vi "ParseArgumentsCore.vi"(8 "error in (no error)":errorcluster, 10 "Inputs":string[](array[string]), 11 "RunVIAnalyzer in":refnum<class "RunVIAnalyzer.lvclass">) -> (0 "error out":errorcluster, 3 "RunVIAnalyzer out":refnum<class "RunVIAnalyzer.lvclass">)   [LabVIEW 2018, in "RunVIAnalyzer.lvclass"]
uses:
  RunVIAnalyzer.lvclass
  RunVIAnalyzer.lvclass/RunVIAnalyzer.ctl
  Utilities/OperationErrorType.ctl
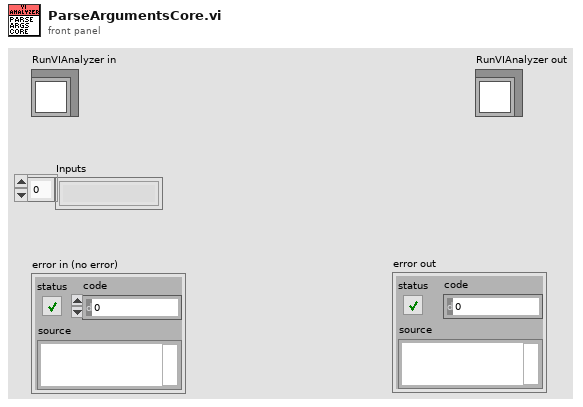
[diagram p1: front panel]
types:
  T1 = typedef "OperationErrorType.ctl" = enum16{"RequiredArgumentMissing", "UnknownArguments", "LoggerSetMultipleTimes", "OperationBrokenError"}
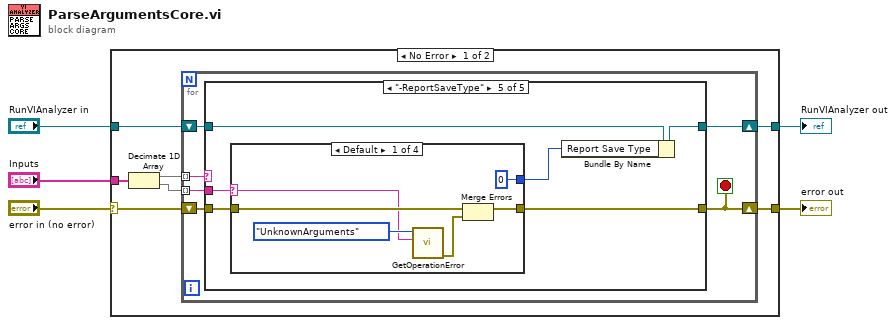
[diagram p0: block diagram]
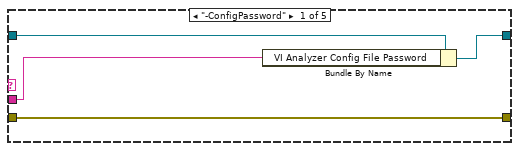
[diagram p2: hidden frame]
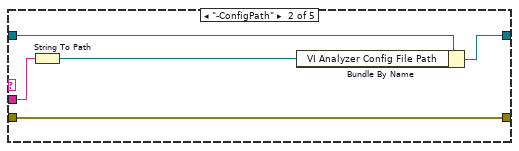
[diagram p3: hidden frame]
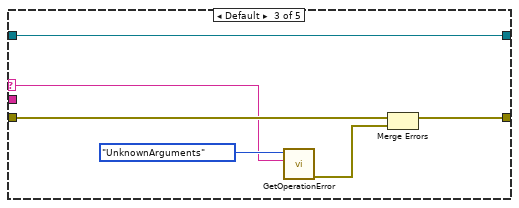
[diagram p4: hidden frame]
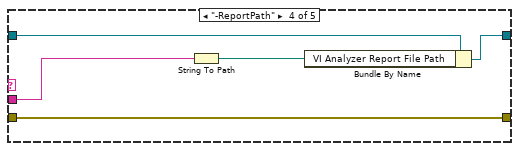
[diagram p5: hidden frame]
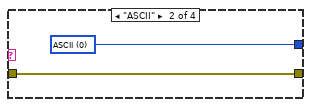
[diagram p6: hidden frame]
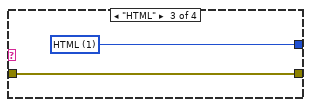
[diagram p7: hidden frame]
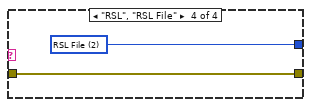
[diagram p8: hidden frame]
diagram:
  n1 = case shown="No Error" "error in (no error)" {
    selector: "error in (no error)" -> [w11 w57]
    tunnel: [w12 w57] -> w5
    tunnel: "Inputs" -> [w8 _]
    tunnel: [w7 w58] -> w2
    tunnel: "RunVIAnalyzer in" -> [w6 w58]
    frame No Error {
      n2 = Decimate 1D Array(w8) -> (w9:string[], w10:string[])
      n3 = for {
        tunnel: w9 -> [w18] mode=indexing
        tunnel: w10 -> [w17] mode=indexing
        shift-right: [w15] -> w7
        shift-left: w6 -> [w16]
        shift-right: [w13] -> w12
        shift-left: w11 -> [w14]
        stop <- w13 stop-if-true
        n4 = case shown="\"-ReportSaveType\"" w18 {
          selector: w18 -> [_ _ w28 _ _]
          tunnel: w17 -> [w19 w25 _ w37 w41]
          tunnel: w16 -> [w22 w27 w33 w38 w44]
          tunnel: [w21 w26 w33 w35 w43] -> w15
          tunnel: w14 -> [w20 w24 w31 w34 w42]
          tunnel: [w20 w24 w29 w34 w40] -> w13
          frame "-ConfigPassword" {
            n5 = Bundle By Name(cluster=w22, "VI Analyzer Config File Password"=w19) -> (w21:refnum<class "RunVIAnalyzer.lvclass">)
          }
          frame "-ConfigPath" {
            n6 = String To Path(string=w25) -> (path=w23:path)
            n7 = Bundle By Name(cluster=w27, "VI Analyzer Config File Path"=w23) -> (w26:refnum<class "RunVIAnalyzer.lvclass">)
          }
          frame Default {
            n8 = call "GetOperationError.vi"("Additional Information"=w28, "Operation Error Type"=OperationErrorType."UnknownArguments") -> ("error out"=w30:errorcluster)  [unwired: 9 in]
            n9 = Merge Errors(w31, w30) -> (w29:errorcluster)
          }
          frame "-ReportPath" {
            n10 = String To Path(string=w37) -> (path=w36:path)
            n11 = Bundle By Name(cluster=w38, "VI Analyzer Report File Path"=w36) -> (w35:refnum<class "RunVIAnalyzer.lvclass">)
          }
          frame "-ReportSaveType" {
            n12 = case shown="Default" w41 {
              selector: w41 -> [w45 _ _ _]
              tunnel: w42 -> [w49 w52 w54 w56]
              tunnel: [w47 w52 w54 w56] -> w40
              tunnel: [u16 0 ("Report Save Type") w51 w53 w55] -> w39
              frame Default {
                n13 = call "GetOperationError.vi"("Additional Information"=w45, "Operation Error Type"=OperationErrorType."UnknownArguments") -> ("error out"=w48:errorcluster)  [unwired: 9 in]
                n14 = Merge Errors(w49, w48) -> (w47:errorcluster)
              }
              frame "ASCII" {
                w51 = u16 0 items=["ASCII", "HTML", "RSL File"] ("Report Save Type")
              }
              frame "HTML" {
                w53 = u16 1 items=["ASCII", "HTML", "RSL File"] ("Report Save Type")
              }
              frame "RSL", "RSL File" {
                w55 = u16 2 items=["ASCII", "HTML", "RSL File"] ("Report Save Type")
              }
            }
            n15 = Bundle By Name(cluster=w44, "Report Save Type"=w39) -> (w43:refnum<class "RunVIAnalyzer.lvclass">)
          }
        }
      }
    }
    frame Error {
    }
  }
  "error out" <- w5
  "RunVIAnalyzer out" <- w2
